vi "Make Counter Signal.vi"(11 "Node Ptr":T1=18446744073709551615 format="%.0x") -> ()   [LabVIEW 2023, in "J1939 Addon System Explorer.lvlib"]
uses:
  J1939 Addon System Explorer.lvlib
  <vilib>/NI VeriStand/Custom Device API/Custom Device Item Ref.ctl
  Addon Shared/SubVIs/Constants.vi
  Addon Shared/J1939 Addon Shared.lvlib
  SubModules/Frame-Protection-Support/Source/System Explorer/Protection and Counter Support System Explorer.lvlib
  <vilib>/NI VeriStand/Custom Device API/Custom Device API.lvlib
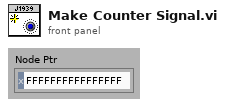
[diagram p1: front panel]
types:
  T1 = typedef "Custom Device API.lvlib/Custom Device Item Ref.ctl" = u64
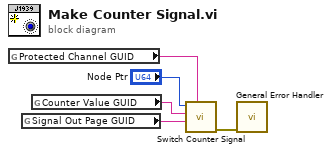
[diagram p0: block diagram]
diagram:
  n1 = global read "Constants.vi" "Protected Channel GUID"() -> (w1:string)
  n2 = global read "Constants.vi" "Signal Out Page GUID"() -> (w3:string)
  n3 = global read "Constants.vi" "Counter Value GUID"() -> (w4:string)
  n4 = call "Switch Counter Signal.vi"("Protected Signal GUID"=w1, "Signal Page GUID"=w3, "Counter Value GUID"=w4, "Node Ptr"="Node Ptr") -> ("error out"=w5:errorcluster)  [unwired: 7 in]
  n5 = call <vilib>:"General Error Handler.vi"("error in (no error)"=w5) -> ()  [unwired: 10 in, 5 out]
